vi "Set IM idle time.vi"(8 "Error In":errorcluster, 9 "Motor index":u8, 10 "IM Idle time":i32, 11 "VISA resource in":refnum<visa-resource-name>) -> (0 "Error Out":errorcluster, 3 "VISA resource out":refnum<visa-resource-name>)   [LabVIEW 2014, in "Motor manager.lvlib"]
uses:
  Motor manager.lvlib
  Typedef/Commands.ctl
  Cmd to Byte Array (Int).vi
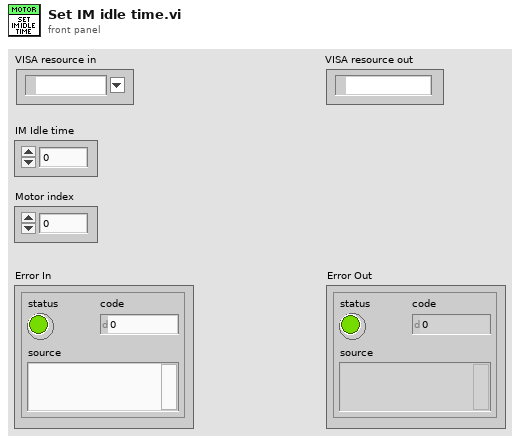
[diagram p1: front panel]
types:
  T1 = typedef "Motor manager.lvlib/Commands.ctl" = enum16{"None", "Set motor", "Set distance", "Set speed", "Set Move Type", "Set IM Idle Time", "Set N cycles", "Start", "Stop", "Stop and Release", "Set Home", "Find Home", "Move Forward", "Move Backward"}
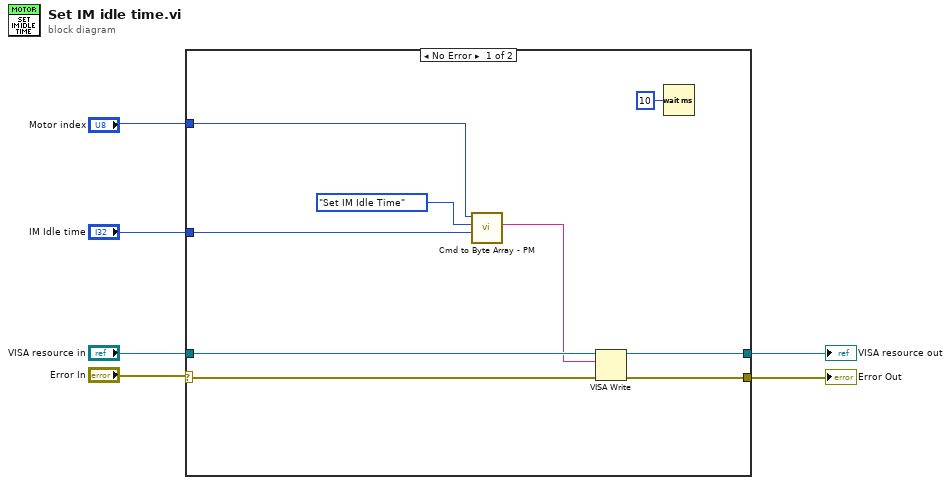
[diagram p0: block diagram]
diagram:
  n1 = case shown="No Error" "Error In" {
    selector: "Error In" -> [w12 w17]
    tunnel: "VISA resource in" -> [w13 w16]
    tunnel: "Motor index" -> [w9 _]
    tunnel: [w15 w17] -> w4
    tunnel: [w14 w16] -> w3
    tunnel: "IM Idle time" -> [w8 _]
    frame No Error {
      n2 = call-poly "Cmd to Byte Array - PM.vi"("Parameter"=w8, "Commands"=Commands."Set IM Idle Time", "Motor index"=w9) -> ("Byte string"=w10:string)  [unwired: 8 in]
      n3 = VISA Write(VISA resource name=w13, write buffer=w10, error in (no error)=w12) -> (VISA resource name out=w14:refnum<visa-resource-name>, error out=w15:errorcluster)  [unwired: 1 out]
      n4 = Wait (ms)(milliseconds to wait=u32 10) -> ()  [unwired: 1 out]
    }
    frame Error {
    }
  }
  "Error Out" <- w4
  "VISA resource out" <- w3
